vi "GetAllErrorsList.vi"(10 "Ftp":refnum<k24>, 11 "error in":errorcluster) -> (2 "Errors":T1(array[cluster]), 3 "error out":errorcluster)   [LabVIEW 2013, in "UnderAutomation.Fanuc.lvlib"]
uses:
  UnderAutomation.Fanuc.lvlib
  C:/Users/fg/Documents/Fanuc.vi/LabVIEW_2024/UnderAutomation.Fanuc/lib/UnderAutomation.Fanuc.dll
  LabVIEW_2024/UnderAutomation.Fanuc/lib/UnderAutomation.Fanuc.dll
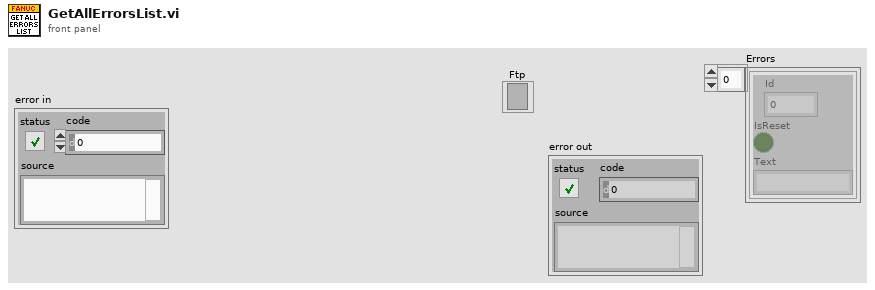
[diagram p1: front panel]
types:
  T1 = cluster{"Id":i32, "IsReset":bool, "Text":string}[]
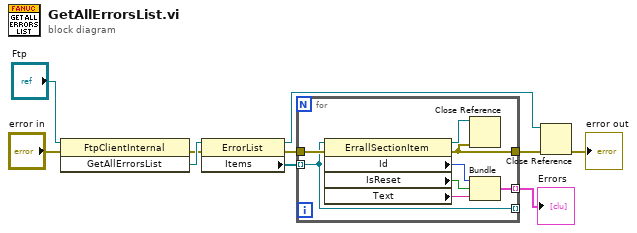
[diagram p0: block diagram]
diagram:
  n1 = invoke class="FtpClientInternal" method="GetAllErrorsList"(reference="Ftp", error in="error in") -> (error out=w7:errorcluster, "GetAllErrorsList"=w8:refnum<k24>)  [unwired: 1 in, 1 out]
  n2 = property class="ErrorList"(reference=w8, error in=w7) -> (reference out=w1:refnum<k24>, error out=w5:errorcluster, "Items"=w6:refnum<k24>[])
  n3 = for {
    tunnel: [w17] -> _ mode=indexing
    tunnel: w5 -> [w18]
    tunnel: [w12] -> w3
    tunnel: w6 -> [w17] mode=indexing
    tunnel: [w13] -> w4 mode=indexing
    n4 = property class="ErrallSectionItem"(reference=w17, error in=w18) -> (reference out=w11:refnum<k24>, error out=w12:errorcluster, "Id"=w16:i32, "IsReset"=w15:bool, "Text"=w14:string)
    n5 = Close Reference(reference=w11, error in (no error)=w12) -> ()  [unwired: 1 out]
    n6 = Bundle("Id"=w16, "IsReset"=w15, "Text"=w14) -> (w13:cluster{"Id":i32, "IsReset":bool, "Text":string})  [unwired: 1 in]
  }
  "Errors" <- w4
  n7 = Close Reference(reference=w1, error in (no error)=w3) -> (error out=→"error out":errorcluster)
